vi "load_timetrace.vi"(8 "Timetraces":T1(array[cluster]), 9 "path in":path, 10 "WaveformGraph in":refnum<vi>, 11 "Last Mouse Position":cluster{"X":i32, "Y":i32}) -> ()   [LabVIEW 2012]
uses:
  <vilib>/Utility/file.llb/Read From Spreadsheet File (DBL).vi
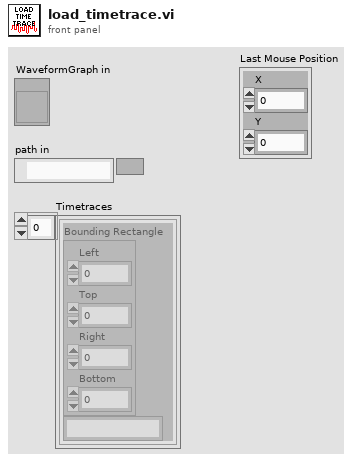
[diagram p1: front panel]
types:
  T1 = cluster{"Bounding Rectangle":cluster{"Left":i32, "Top":i32, "Right":i32, "Bottom":i32}, string}[]
  T2 = cluster{"Left":i32, "Top":i32, "Right":i32, "Bottom":i32}
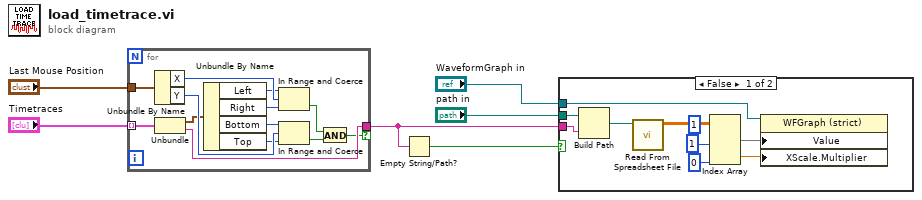
[diagram p0: block diagram]
diagram:
  n1 = for {
    tunnel: "Timetraces" -> [w19] mode=indexing
    tunnel: "Last Mouse Position" -> [w18]
    tunnel: [w9] -> w5 if=w7
    n2 = Unbundle By Name(w18) -> ("X"=w17:i32, "Y"=w14:i32)
    n3 = Unbundle(w19) -> ("Bounding Rectangle"=w8:T2, w9:string)
    n4 = Unbundle By Name(w8) -> ("Left"=w16:i32, "Right"=w15:i32, "Bottom"=w13:i32, "Top"=w12:i32)
    n5 = In Range and Coerce(upper limit=w16, x=w17, lower limit=w15) -> (In Range?=w11:bool)  [unwired: 1 out]
    n6 = In Range and Coerce(upper limit=w13, x=w14, lower limit=w12) -> (In Range?=w10:bool)  [unwired: 1 out]
    n7 = And(x=w11, y=w10) -> (x .and. y?=w7:bool)
  }
  n8 = Empty String/Path?(string/path=w5) -> (empty?=w6:bool)
  n9 = case shown="False" w6 {
    tunnel: "path in" -> [w26 _]
    tunnel: w5 -> [w25 _]
    tunnel: "WaveformGraph in" -> [w23 _]
    frame False {
      n10 = Build Path(base path=w26, name or relative path=w25) -> (appended path=w27:path)
      n11 = call-poly <vilib>:"Read From Spreadsheet File.vi"("file path (dialog if empty)"=w27) -> ("all rows"=w28:dbl[][])  [unwired: 6 in, 4 out]
      n12 = Index Array(array=w28, index (col) #1=1 ("disabled index (col)"), index (row) #2=1 ("disabled index (row)"), index (col) #2=0 ("index (col)")) -> (element #1=w24:dbl[], element #2=w20:dbl)  [unwired: 1 in]
      n13 = property class="WFGraph (strict)"(reference=w23, "Value"=w24, "XScale.Multiplier"=w20) -> ()  [unwired: 1 in, 2 out]
    }
    frame True {
    }
  }
